vi "Start.vi"(8 "error in (no error)":errorcluster, 10 "Params":variant, 11 "PmuDelayClass in":refnum<class "PmuDelay.lvclass">) -> (0 "error out":errorcluster, 3 "PmuDelayClass out":refnum<class "PmuDelay.lvclass">)   [LabVIEW 2018, in "AnalysisPlugins.lvlib" / "PmuDelay.lvclass"]
uses:
  PmuDelay.lvclass
  C:/projects/ICDAS/NistPluggableModules/Analysis/AnalysisPlugins/AnalysisPluginBaseClass/AnalysisPluginsBase.lvclass
  C:/projects/ICDAS/NistPluggableModules/Analysis/AnalysisPlugins/FitterBaseClass/FitterBase.lvclass
  C:/projects/ICDAS/NistPluggableModules/Analysis/AnalysisPlugins/PmuAnalysisClass/PmuAnalysis.lvclass
  FGen/MemberClasses/PmuTestFunctions/Typedefs/PmuTestParams.ctl
  PmuAnalysisClass/PmuAnalysis.lvclass/PmuAnalysis.ctl
  FGen/MemberClasses/PmuTestFunctions/Typedefs/eParamIdx.ctl
  AnalysisPluginBaseClass/AnalysisPluginsBase.lvclass/AnalysisPluginsBase.ctl
  PmuAnalysisClass/Accessors/Read eTestType.vi
  AnalysisPluginBaseClass/Accessors/Write FileName.vi
  <vilib>/Utility/error.llb/Error Cluster From Error Code.vi
  <vilib>/ErrorRing/Error Ring.xnode
  FGen/MemberClasses/PmuTestFunctions/PmuTestFunctions.lvclass
  PmuAnalysisClass/PmuAnalysis.lvclass
  AnalysisPluginBaseClass/AnalysisPluginsBase.lvclass
  FitterBaseClass/FitterBase.lvclass
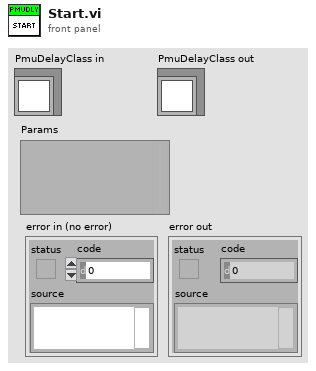
[diagram p1: front panel]
types:
  T1 = typedef "Functions.lvlib/PmuTestFunctions.lvclass/PmuTestParams.ctl" = dbl[][]
  T2 = typedef "Functions.lvlib/PmuTestFunctions.lvclass/eParamIdx.ctl" = enum16{"Xm", "Fin", "Ps", "Fh", "Ph", "Kh", "Fa", "Ka", "Fx", "Kx", "Rf", "KaS", "KxS", "KfS", "KrS"}
  T3 = enum16{"SteadyState", "Modulation", "Ramp", "Step"}
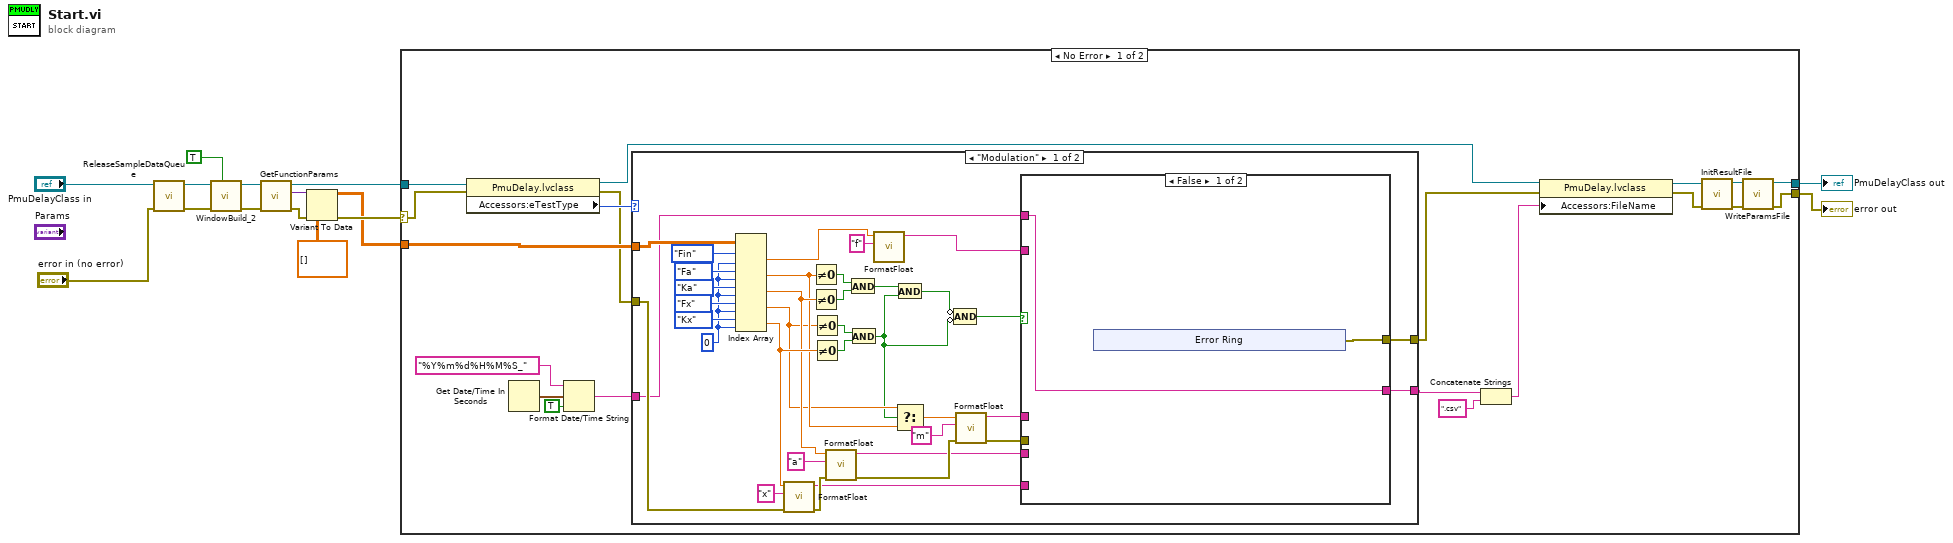
[diagram p0: block diagram]
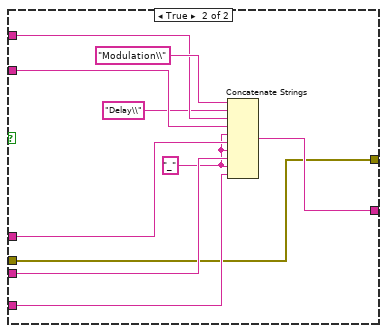
[diagram p2: hidden frame]
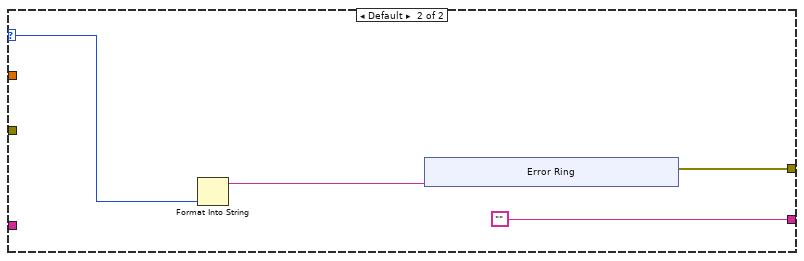
[diagram p3: hidden frame]
diagram:
  n1 = call "ReleaseSampleDataQueue.vi"("error in (no error)"="error in (no error)", "AnalysisPluginsBase in"="PmuDelayClass in") -> ("error out"=w6:errorcluster, "AnalysisPluginsBase out"=w5:refnum<class "PmuDelay.lvclass">)  [unwired: 8 in]
  n2 = call "WindowBuild_2.vi"("Init"=TRUE, "Error In"=w6, "Fitter in"=w5) -> ("Error Out"=w3:errorcluster, "Fitter out"=w4:refnum<class "PmuDelay.lvclass">)  [unwired: 6 in, 1 out]
  n3 = call-dynamic "GetFunctionParams.vi"("error in (no error)"=w3, "PmuAnalysis in"=w4) -> ("error out"=w14:errorcluster, "FunctionParams"=w15:variant, "PmuAnalysis out"=w11:refnum<class "PmuDelay.lvclass">)  [unwired: 7 in]
  n4 = Variant To Data(error in=w14, type=T1 [] ("Accessors:PmuTestParams"), Variant=w15) -> (data=w10:T1, error out=w12:errorcluster)
  n5 = case shown="No Error" w12 {
    selector: w12 -> [w34 w100]
    tunnel: w11 -> [w35 w101]
    tunnel: w10 -> [w29 _]
    tunnel: [w17 w101] -> w2
    tunnel: [w16 w100] -> w9
    frame No Error {
      n6 = property class="PmuDelay.lvclass"(reference=w35, error in=w34) -> (reference out=w26:refnum<class "PmuDelay.lvclass">, error out=w28:errorcluster, "Accessors:eTestType"=w30:T3)
      n7 = Get Date/Time In Seconds() -> (seconds since 1Jan1904=w32:timestamp)
      n8 = Format Date/Time String(time format string (%c)="%Y%m%d%H%M%S_", seconds (now)=w32, UTC format=TRUE) -> (date/time string=w27:string)
      n9 = case shown="\"Modulation\"" w30 {
        selector: w30 -> [_ w91]
        tunnel: w28 -> [w59 _]
        tunnel: w29 -> [w71 _]
        tunnel: w27 -> [w56 _]
        tunnel: [w50 ""] -> w23
        tunnel: [w36 w90] -> w25
        frame "Modulation" {
          w49 = 0 ("disabled index (col)")
          n10 = Index Array(array=w71, index (row) #1=eParamIdx."Fin" ("eParamIdx"), index (col) #1=w49, index (row) #2=eParamIdx."Fa" ("eParamIdx"), index (col) #2=w49, index (row) #3=eParamIdx."Ka" ("eParamIdx"), index (col) #3=w49, index (row) #4=eParamIdx."Fx" ("eParamIdx"), index (col) #4=w49, index (row) #5=eParamIdx."Kx" ("eParamIdx"), index (col) #5=w49) -> (element #1=w45:dbl, element #2=w42:dbl, element #3=w47:dbl, element #4=w41:dbl, element #5=w60:dbl)
          n11 = call "FormatFloat.vi"("error in (no error)"=w59, "replace string (\".\")"="x" ("replace string (\".\")"), "float"=w60) -> ("error out"=w57:errorcluster, "string"=w51:string)  [unwired: 7 in]
          n12 = Not Equal To 0?(x=w42) -> (x != 0?=w65:bool)
          n13 = Not Equal To 0?(x=w47) -> (x != 0?=w66:bool)
          n14 = Not Equal To 0?(x=w41) -> (x != 0?=w64:bool)
          n15 = Not Equal To 0?(x=w60) -> (x != 0?=w63:bool)
          n16 = call "FormatFloat.vi"("error in (no error)"=w57, "replace string (\".\")"="a" ("replace string (\".\")"), "float"=w47) -> ("error out"=w53:errorcluster, "string"=w52:string)  [unwired: 7 in]
          n17 = And(x=w65, y=w66) -> (x .and. y?=w62:bool)
          n18 = And(x=w64, y=w63) -> (x .and. y?=w39:bool)
          n19 = call "FormatFloat.vi"("replace string (\".\")"="f" ("replace string (\".\")"), "float"=w45) -> ("string"=w43:string)  [unwired: 8 in, 1 out]
          n20 = And(x=w62, y=w39) -> (x .and. y?=w40:bool)
          n21 = Select(t=w41, s=w39, f=w42) -> (s? t:f=w55:dbl)
          n22 = Compound Arithmetic op=AND(invert w40, invert w39) -> (w38:bool)
          n23 = call "FormatFloat.vi"("error in (no error)"=w53, "replace string (\".\")"="m" ("replace string (\".\")"), "float"=w55) -> ("error out"=w37:errorcluster, "string"=w44:string)  [unwired: 7 in]
          n24 = case shown="False" w38 {
            tunnel: w56 -> [w72 w87]
            tunnel: w52 -> [_ w86]
            tunnel: w51 -> [_ w85]
            tunnel: [w72 w84] -> w50
            tunnel: w44 -> [_ w83]
            tunnel: w43 -> [_ w82]
            tunnel: w37 -> [_ w79]
            tunnel: [w73 w79] -> w36
            frame False {
              n25 = xnode "Error Ring"() -> ("error out"=w73:errorcluster)
            }
            frame True {
              w81 = "_" ("string")
              n26 = Concatenate Strings("Modulation\\", "Delay\\", w87, w82, w81, w83, w81, w86, w81, w85) -> (w84:string)
            }
          }
        }
        frame Default {
          n27 = Format Into String(w91) -> (resulting string=w92:string)  [unwired: 3 in, 1 out]
          n28 = xnode "Error Ring"("parameter 0"=w92) -> ("error out"=w90:errorcluster)
        }
      }
      n29 = Concatenate Strings(w23, ".csv" ("string")) -> (w22:string)
      n30 = property class="PmuDelay.lvclass"(reference=w26, error in=w25, "Accessors:FileName"=w22) -> (reference out=w21:refnum<class "PmuDelay.lvclass">, error out=w20:errorcluster)
      n31 = call-dynamic "InitResultFile.vi"("error in (no error)"=w20, "PmuDelayClass in"=w21) -> ("error out"=w18:errorcluster, "PmuDelayClass out"=w19:refnum<class "PmuDelay.lvclass">)  [unwired: 8 in]
      n32 = call "WriteParamsFile.vi"("error in (no error)"=w18, ":PmuAnalysis"=w19) -> ("error out"=w16:errorcluster, "PmuAnalysis"=w17:refnum<class "PmuDelay.lvclass">)  [unwired: 8 in]
    }
    frame Error {
    }
  }
  "error out" <- w9
  "PmuDelayClass out" <- w2
